vi "332 Range Set.vi"(0 "Power Range: 93C\n0=OFF, 1=Low, 2=Med, 3=High":sgl) -> ()   [LabVIEW 2012]
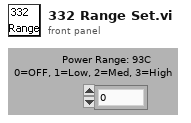
[diagram p1: front panel]
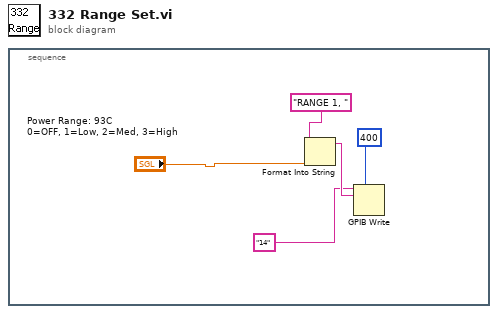
[diagram p0: block diagram]
diagram:
  n1 = stacked-sequence {
    frame #0 {
      n2 = Format Into String(initial string="RANGE 1, ", "Power Range: 93C\n0=OFF, 1=Low, 2=Med, 3=High") -> (resulting string=w5:string)  [unwired: 2 in, 1 out]
      n3 = GPIB Write(0:"14", 1:w5, 4:400) -> ()  [unwired: 2 in, 2 out]
    }
  }
